vi "Dashboard Main.vi"() -> ()   [LabVIEW 2019]
uses:
  <vilib>/event_ctls.llb/eventvkey.ctl
  <vilib>/Rock Robotics/WPI/Dashboard/WPI_DashboardLogging Global.vi
  <vilib>/Utility/miscctls.llb/LVRowAndColumnTypeDef.ctl
  UnderControl2020/Corsair_V2/Team Code/MotorsGlobal.vi
  UnderControl2020/Corsair_V1/Team Code/Climber Routine.ctl
  <vilib>/Rock Robotics/Network Tables/NT Read Boolean.vi
  UnderControl2020/Corsair_V2/Team Code/JoysticksGlobal.vi
  <vilib>/Rock Robotics/Network Tables/NT Read Numeric Array.vi
  <vilib>/Rock Robotics/Network Tables/NT Read Variant.vi
panel:
  in  "Camera Settings Right":T1={"Frame Rate"=30, "Compression"=30, "Size"=1, "DB Camera Config"=FALSE} {"Frame Rate" scale=1.0..30.0; "Compression" scale=100.0..-1.0; "Size" items=["640x480", "320x240", "160x120"]}
  in  "Camera Name Right":string(combo)="No Camera Selection"
  out "Camera Perf":string
  in  "Camera Settings":T1={"Frame Rate"=30, "Compression"=30, "Size"=1, "DB Camera Config"=FALSE} {"Frame Rate" scale=1.0..30.0; "Compression" scale=100.0..-1.0; "Size" items=["640x480", "320x240", "160x120"]}
  in  "TCP":refnum<k5>
  in  "Rec Mode":enum32{"Stop", "Record", "Playback"}(radio)
  out "Robot IP":string
  out "Image Message":string="Timeout in Camera Communications"
  in  "Dashboard Tab":T2(tab)
  in  "Select Auto":string(combo)="Select Autonomous ..."
  out "NT Connection":bool
  out "MotorChart R":cluster{"Numeric":dbl, "Numeric":dbl}(graph)
  out "MotorChart L":cluster{"Numeric":dbl, "Numeric":dbl}(graph)
  out "MotorSliders R":cluster{"MotorSlide1":dbl, "MotorSlide2":dbl} {"MotorSlide2" scale=-1.0..1.0 scale format="%#_2e"; "MotorSlide1" scale=-1.0..1.0 scale format="%#_2e"}
  out "MotorSliders L":cluster{"MotorSlide1":dbl, "MotorSlide2":dbl} {"MotorSlide2" scale=-1.0..1.0 scale format="%#_2e"; "MotorSlide1" scale=-1.0..1.0 scale format="%#_2e"}
  out "Gyro":dbl(knob) scale=0.0..360.0
  out "JS1 Z":dbl(slide) scale=-1.0..1.0 scale format="%#_2e"
  out "JS1 Graph":cluster{"X":dbl, "Y":dbl}[](graph)
  out "JS1 Buttons":T3
  out "JS2 Z":dbl(slide) scale=-1.0..1.0 scale format="%#_2e"
  out "JS2 Graph":cluster{"X":dbl, "Y":dbl}[](graph)
  out "JS2 Buttons":T3
  out "Mode":T4(ring)=enum."Auto Disabled"
  out "Right Camera Perf":cluster{"Bandwidth (Mbps)":dbl, "FPS":dbl}
  out "Intake on?":bool
  out "LL Valid Target?":bool
  out "Conveyor IR":bool
  out "Climber on?":bool
  out "PTO activated?":bool
  out "Shooter Mode":string
  out "Limelight X":dbl
  out "LimelightY":dbl
  out "Pra qual lado?":string
  out "Camera Image Right":T5(plugin-control)
  in  "DB/String 9":string
  in  "DB/String 8":string
  in  "DB/String 7":string
  in  "DB/String 6":string
  in  "DB/String 5":string
  in  "DB/String 4":string
  in  "DB/String 3":string
  in  "DB/String 2":string
  in  "DB/String 1":string
  in  "DB/String 0":string
  in  "DB/Slider 0":dbl(slide) scale=0.0..5.0
  in  "DB/Slider 1":dbl(slide) scale=0.0..5.0
  in  "DB/Slider 2":dbl(slide) scale=0.0..5.0
  in  "DB/Slider 3":dbl(slide) scale=0.0..5.0
  out "DB/LED 3":bool
  out "DB/LED 2":bool
  out "DB/LED 1":bool
  out "DB/LED 0":bool
  in  "DB/Button 3":bool
  in  "DB/Button 2":bool
  in  "DB/Button 1":bool
  in  "DB/Button 0":bool caption="New Name"
  out "LL Valid Target?.":bool
  out "FlywheelSetpoint":dbl
  out "Reset Encoder":bool
  out "LL in Range?":bool
  out "ClimberSolenoid":bool
  out "LL Mode":dbl
  out "LL LED Status":dbl
  out "TurretEncoder":dbl
  out "RollerOutput":dbl
  out "ConveyorRight\nOutput":dbl
  out "CoveyorLeft\nOutput":dbl
  out "ConveyorMid\nOutput":dbl
  out "IntakeOutput":dbl
  out "ClimberOutput":dbl
  out "Climber on?.":bool
  out "Limelight X 2":dbl
  out "LimelightY 2":dbl
  out "PTO activated?.":bool
  out "Conveyor IR.":bool
  out "Intake on?.":bool
  out "Rumble":dbl
  out "Shooter Mode.":string
  in  "Test Slider":dbl(slide) scale=0.0..100.0 scale format="%#_3g"
  in  "On/Off":bool caption="Solenoid"
  in  "Test Name":u16(ring) items=["Select the test to run..."]
  in  "Test Tree":string(tree)
  in  "Motor":cluster{"Value":dbl, "Enable":bool} {"Value" scale=-1.0..1.0 scale format="%#_3g"}
  out "Progress":T6 {"Test Progress" scale=0.0..100.0}
  in  "Rev/Fwd":cluster{"Forward":bool, "Reverse":bool}
  in  "Test Ring":u16(ring) items=["Monochrome", "Color"]
  out "Cmd Status":string
  in  "Execute Command":bool
  in  "Command Params":string[][](table)
  in  "Command Selection":i32(listbox)
  in  "CheckList":i32(listbox)
  out "Tree":string(tree)
  out "Camera Image":T5(plugin-control)
  in  "Camera Name":string(combo)="No Camera Selection"
  # "HW"
  # "HW"
  # "Drive Motors"
  # "Joysticks"
  # "Front"
  # "Left"
  # "Back"
  # "Shooter"
  # "Conveyor and intake"
  # "Climber"
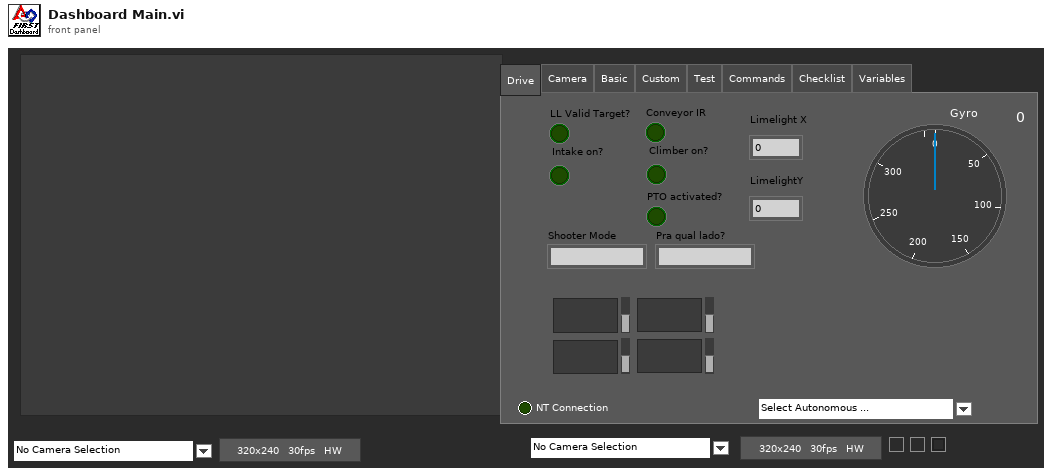
[diagram p1: front panel]
types:
  T1 = cluster{"Frame Rate":i32, "Compression":i32, "Size":u16, "DB Camera Config":bool}
  T2 = enum32{"Drive", "Camera", "Basic", "Custom", "Test", "Commands", "Checklist", "Variables"}
  T3 = cluster{bool, bool, bool, bool, bool, bool, bool, bool, bool, bool, bool, bool}
  T4 = enum8{"Tele-Op Disabled", "Tele-Op Enabled", "Auto Disabled", "Auto Enabled", "Test Disabled", "Test Enabled", "Disconnected", "No Code", "E-Stop"}
  T5 = typedef "IMAQ Image.ctl" = refnum<image>
  T6 = cluster{"Test Progress":u8, "Test Progress Text":string}
  T7 = cluster{"Save Path":path, "Interval (s)":dbl, "Keep":i32}
  T8 = typedef "Image Type" = u32
  T9 = cluster{"IDs":cluster{"RPC field ID":u16, "Unique ID":u16}, "String":string}
  T10 = typedef "Climber Routine.ctl" = enum16{"Standart", "Vibrate *Lenny Face*", "Open da Boi", "Engage on the Bar!", "Pull Our Hope", "Deu por Hoje"}
  T11 = cluster{"Error Strings":string, "Disable Counts":cluster{u16, u16}, "Rail Faults":cluster{u16, u16, u16}, "Robot IP":string, "DB Mode":u8, "Event Info":cluster{"Name":string, "Type":u8, "Number":u16, "Replay":u8}}
  T12 = cluster{"Storage":cluster{"Disk Free":u64, "RAM Block":u32, "RAM free":u32}, "CPU Utilization":cluster{"CPU % ISR":sgl, "CPU % Time Crit":sgl, "CPU % Timed Str":sgl, "CPU % High":sgl, "CPU % Above":sgl, "CPU % Normal":sgl, "CPU % Low":sgl}, "CAN":cluster{"% Bus Utilization":sgl, "Bus Off Cnt":u32, "TX_FIFO Full Cnt":u32, "Receive Error Cnt":u8, "Transmit Error Cnt":u8}, "HID":cluster{"HID Outputs":u32, "Rumble Low":u16, "Rumble High":u16}[]}
  T13 = cluster{"Status bits":cluster{"Test Mode":bool, "Autonomous":bool, "Enabled":bool, "Code Start":bool, "Brownout":bool, "Reserved 2":bool, "Reserved 3":bool, "E-Stop":bool}, "Code Trace":cluster{"Disabled":bool, "TeleOp":bool, "Auto":bool, "Test":bool}, "Controller Type":enum16{"unknown", "cRIO", "roboRio"}, "Code?":enum16{"unknown", "noCode", "code"}, "Battery V":dbl}
  T14 = cluster{"Control Bits":cluster{"TestMode":bool, "Autonomous":bool, "Enabled":bool, "FMS Present":bool, bool, bool, bool, "E-Stop":bool}, "Team Station ":u8, "Countdown":sgl, "Joystick Values":cluster{"Axes":dbl[], "Buttons":bool[], "POVs":i16[]}[]}
  T15 = cluster{"Axes":dbl[], "Buttons":bool[], "POVs":i16[]}[]
  T16 = cluster{"Axes":dbl[], "Buttons":bool[], "POVs":i16[]}
  T17 = cluster{"Buttons[0]":bool, "Buttons[1]":bool, "Buttons[2]":bool, "Buttons[3]":bool, "Buttons[4]":bool, "Buttons[5]":bool, "Buttons[6]":bool, "Buttons[7]":bool, "Buttons[8]":bool, "Buttons[9]":bool, "Buttons[10]":bool, "Buttons[11]":bool}
  T18 = cluster{"Camera Image":refnum<vi>, "Dashboard Tab":refnum<vi>, void, "Rec Mode":refnum<vi>, "Test Slider":refnum<vi>, "On/Off ":refnum<vi>, "Test Ring":refnum<vi>, "Rev/Fwd":refnum<vi>, "Test Name":refnum<vi>, "Motor":refnum<vi>, "Progress":refnum<vi>, "CheckList":refnum<vi>, "Tree":refnum<vi>, "Test Tree":refnum<vi>, "Command Params":refnum<vi>, "Command Selection":refnum<vi>, "Execute Command":refnum<vi>, "Cmd Status":refnum<vi>, "Camera Settings":refnum<vi>, "Camera Name":refnum<vi>, "Camera Perf":refnum<vi>, "Camera Settings Right":refnum<vi>, "Camera Name Right":refnum<vi>, "Camera Image Right":refnum<vi>}
  T19 = cluster{"Global Rectangle":i32[], "Contours":cluster{"Contour Type":u32, "ROI Type":u32, "Points":i32[]}[]}
  T20 = cluster{"Camera Name":string, string, "Saved DB Images Info":cluster{"Save Path":path, "Interval (s)":dbl, "Keep":i32}}
  T21 = cluster{"Camera Name Right":string, string, "Saved DB Images Info":cluster{"Save Path":path, "Interval (s)":dbl, "Keep":i32}}
  T22 = cluster{"Operation":enum16{"Update", "Clear"}, "Color Box":u32}[]
  T23 = typedef "eventvkey.ctl" = enum16{"ASCII", "Enter", "Return", "Shift", "Ctrl", "Alt", "Cmd", "Opt", "Caps", "NumLock", "Clear", "Break", "Up", "Down", "Left", "Right", "Insert", "Delete", "Home", "End", "PageUp", "PageDown", "Escape", "Help", "Pause", "ScrollLock", "F1", "F2", "F3", "F4", "F5", "F6", "F7", "F8", "F9", "F10", "F11", "F12", "F13", "F14", "F15", "F16", "F17", "F18", "F19", "F20", "F21", "F22", "F23", "F24", "Play", "VolumeUp", "VolumeDown", "Mute", "Two Byte Char"}
  T24 = cluster{"Image Size":bool, "Image Type":bool, "Pixel Value":bool, "ROI Information":bool, "Zoom Factor":bool}
  T25 = cluster{"Operation":enum16{"Update", "Clear"}, "Color Box":u32}
  T26 = typedef "LVRowAndColumnTypeDef.ctl" = cluster{"Row":i32, "Column":i32}
  T27 = cluster{"Shift":bool, "Ctrl":bool, "Alt":bool, "Cmd":bool, "Opt":bool}
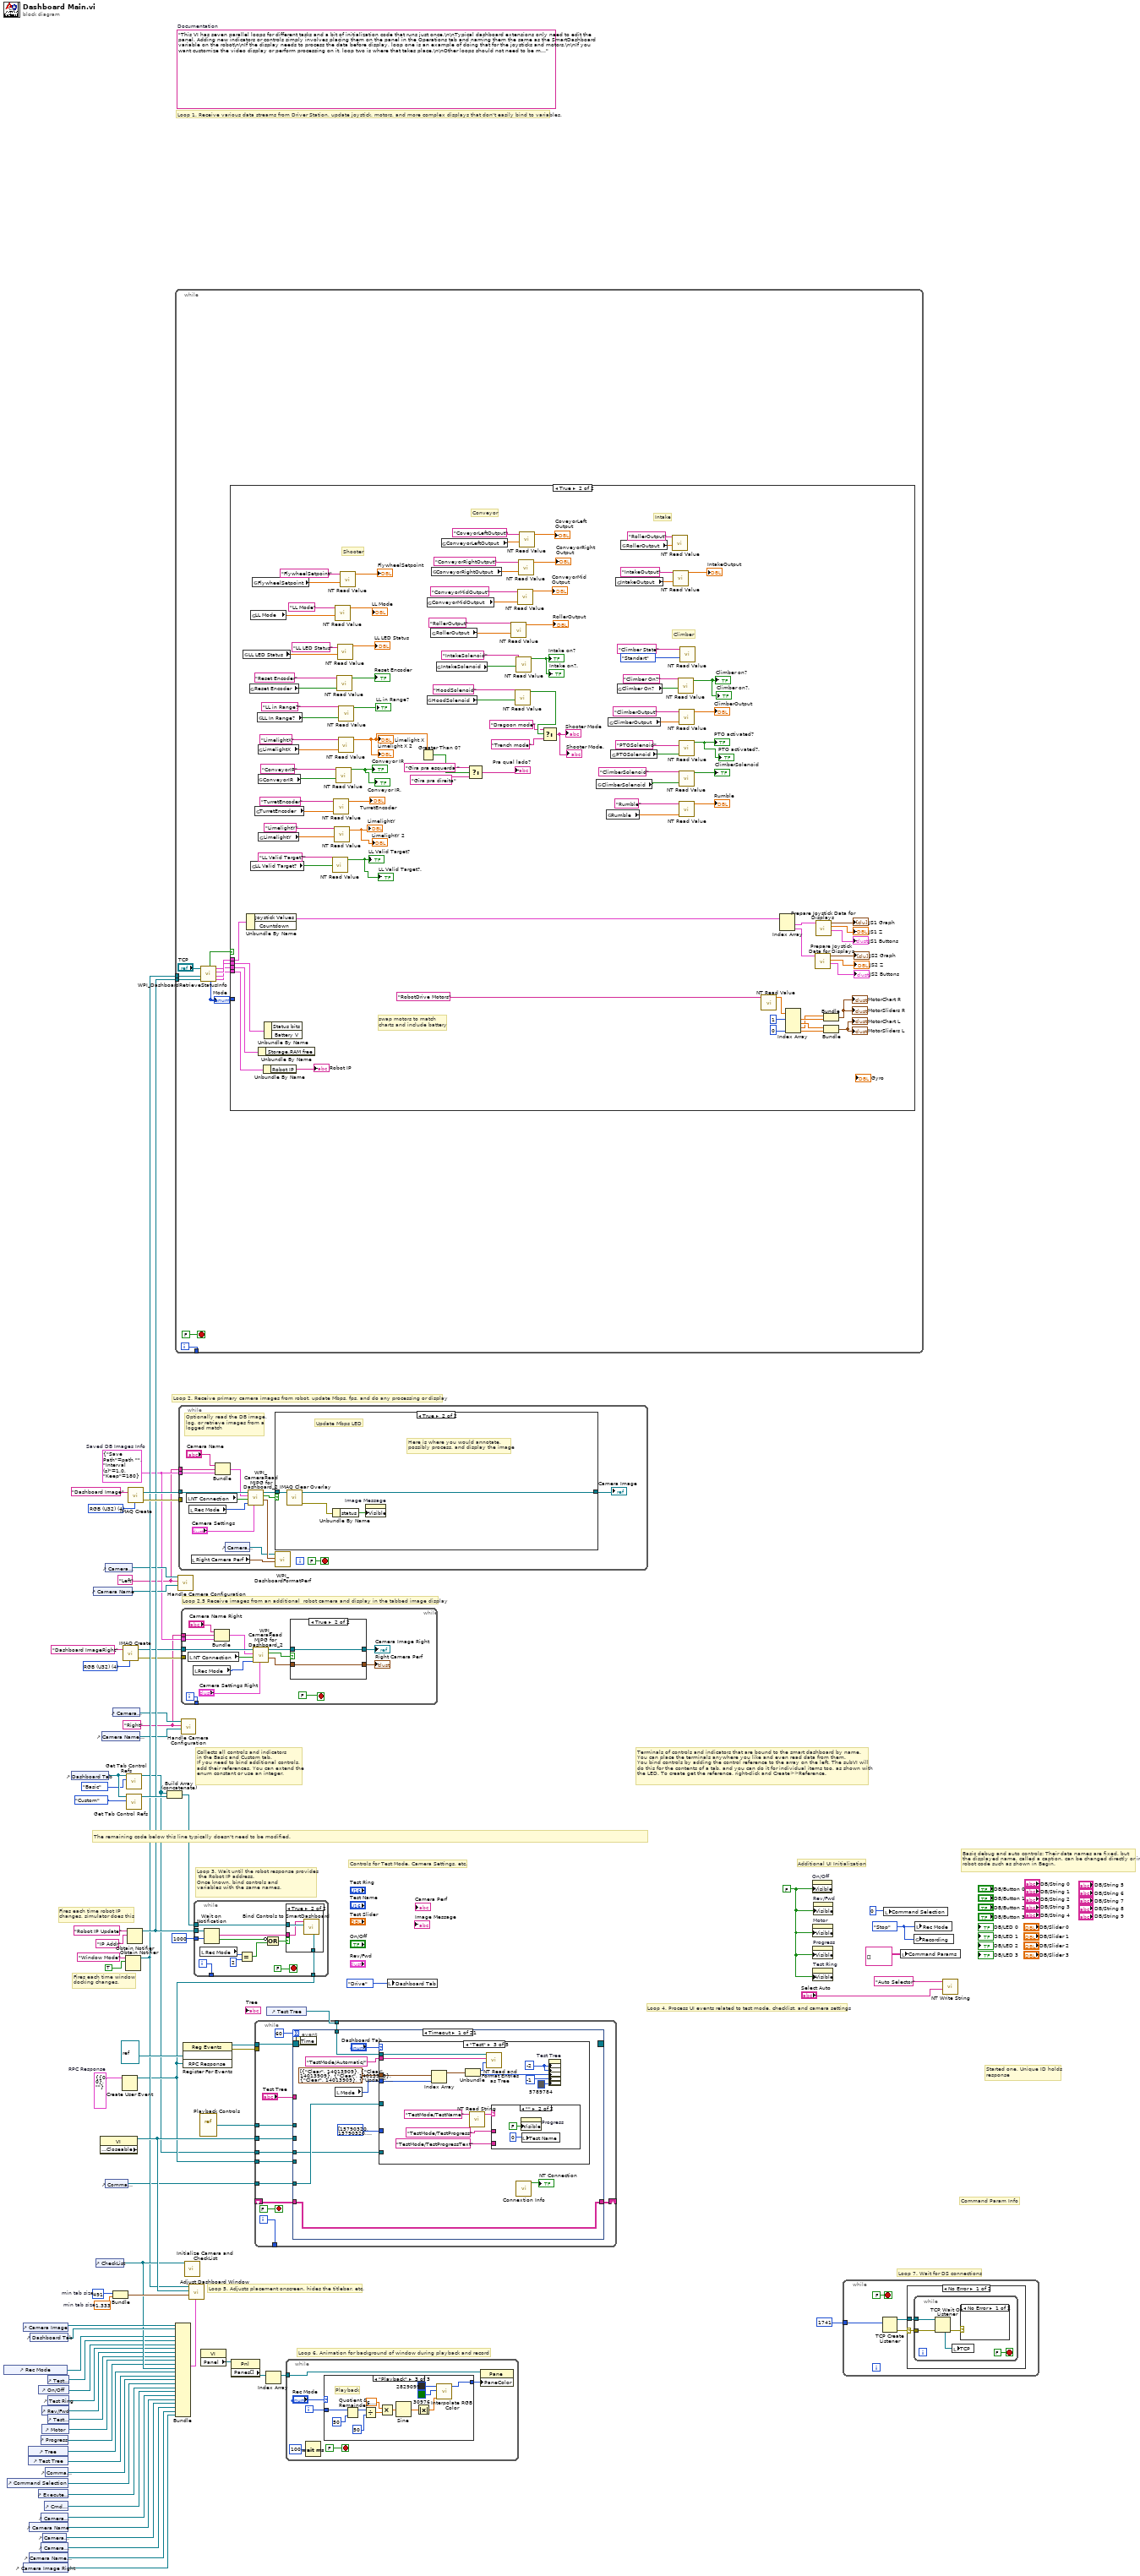
[diagram p0: block diagram]
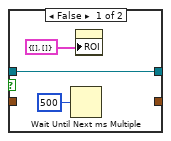
[diagram p2: hidden frame]
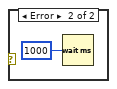
[diagram p3: hidden frame]
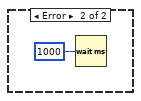
[diagram p4: hidden frame]
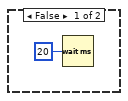
[diagram p5: hidden frame]
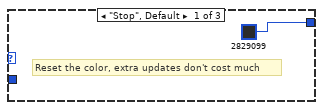
[diagram p6: hidden frame]
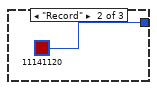
[diagram p7: hidden frame]
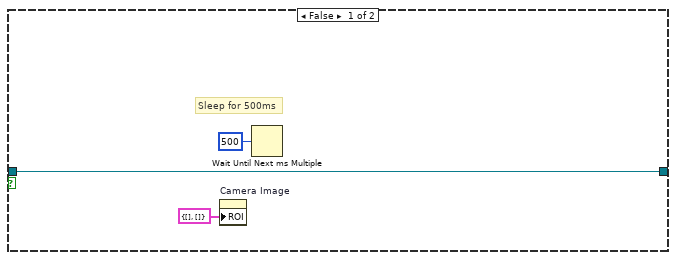
[diagram p9: hidden frame]
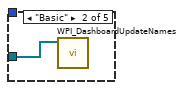
[diagram p11: hidden frame]
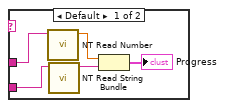
[diagram p12: hidden frame]
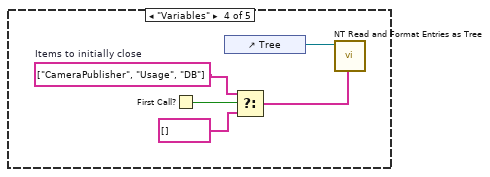
[diagram p13: hidden frame]
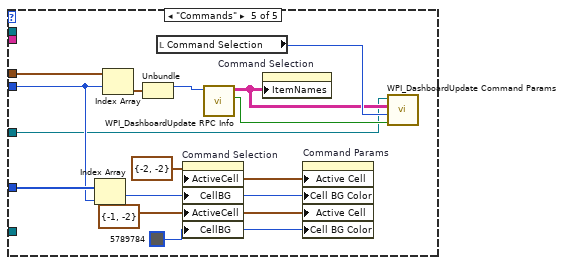
[diagram p14: hidden frame]
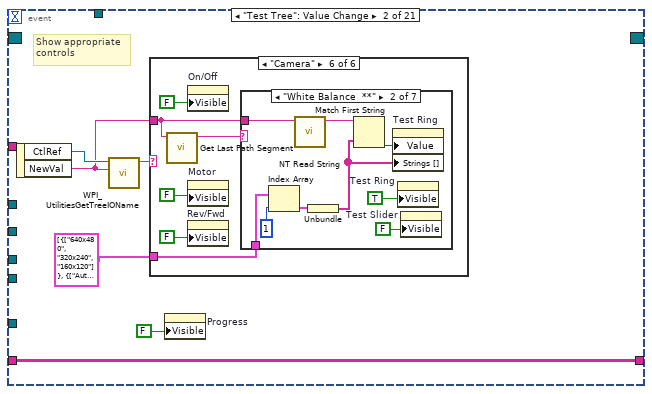
[diagram p15: hidden frame]
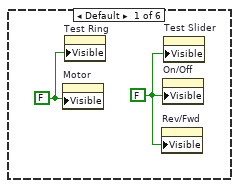
[diagram p16: hidden frame]
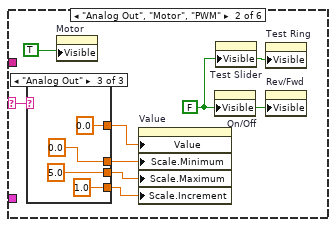
[diagram p17: hidden frame]
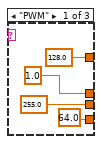
[diagram p18: hidden frame]
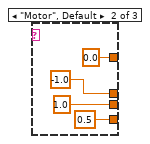
[diagram p19: hidden frame]
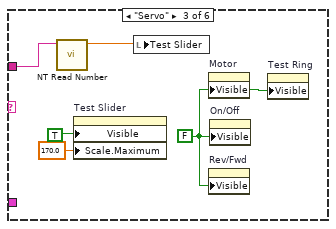
[diagram p20: hidden frame]
diagram:
  w3 = T7 {"Save Path"=path "", "Interval (s)"=1.0, "Keep"=180}  # Saved DB Images Info
  w2 = "Right"
  w1 = "Left"
  w13 = T8 4 items=["Grayscale (U8)", "Grayscale (I16)", "Grayscale (SGL)", "Complex (CSG)", "RGB (U32)", "HSL (U32)", "RGB (U64)"] ("Image Type")
  w29 = T9 {"IDs"={"RPC field ID"=0, "Unique ID"=0}, "String"=""}  # RPC Response
  w52 = 491  # min tab size
  w51 = 1.333  # min tab size
  w59 = enum32{"Stop", "Record", "Playback"}."Stop" ("Rec Mode")
  w36 = FALSE ("Visible")
  (unwired) "This VI has seven parallel loops for different tasks and a bit of initialization code that runs just once.\n\nTypical dashboard extensions only need to edit the panel. Adding new indicators or controls simply involves placing them on the panel in the Operations tab and naming them the same as the SmartDashboard variable on the robot\n\nIf the display needs to process the data before display, loop one is an example of doing that for the joysticks and motors.\n\nIf you want customize the video display or perform processing on it, loop two is where that takes place.\n\nOther loops should not need to be modified. They are pretty standard, and document the task they perform."  # Documentation
  w76 = T8 4 items=["Grayscale (U8)", "Grayscale (I16)", "Grayscale (SGL)", "Complex (CSG)", "RGB (U32)", "HSL (U32)", "RGB (U64)"] ("Image Type")
  # "Loop 2.5 Receive images from an additional  robot camera and display in the tabbed image display"
  # "Command Param Info"
  # "Started one, Unique ID holds\nresponse"
  # "Loop 7. Wait for DS connections"
  # "Basic debug and auto controls: Their data names are fixed, but\nthe displayed name, called a caption, can be changed directly or in\nrobot code such as shown in Begin."
  # "Controls for Test Mode, Camera Settings, etc."
  # "Additional UI Initialization"
  # "Loop 6. Animation for background of window during playback and record"
  # "Fires each time robot IP\nchanges, simulator does this"
  # "Fires each time window\ndocking changes."
  # "Collects all controls and indicators\nin the Basic and Custom tab.\nIf you need to bind additional controls,\nadd their references. You can extend the\nenum constant or use an integer."
  # "The remaining code below this line typically doesn't need to be modified."
  # "Loop 4. Process UI events related to test mode, checklist, and camera settings"
  # "Terminals of controls and indicators that are bound to the smart dashboard by name.\nYou can place the terminals anywhere you like and even read data from them.\nYou bind controls by adding the control reference to the array on the left. The subVI will\ndo this for the contents of a tab, and you can do it for individual items too, as shown with\nthe LED. To create get the reference, right-click and Create>>Reference."
  # "Loop 3. Wait until the robot response provides\n the Robot IP address.\nOnce known, bind controls and\nvariables with the same names."
  # "Loop 5. Adjusts placement onscreen, hides the titlebar, etc."
  # "Loop 1. Receive various data streams from Driver Station, update joystick, motors, and more complex displays that don't easily bind to variables."
  # "Loop 2. Receive primary camera images from robot, update Mbps, fps, and do any processing or display"
  n1 = control-ref of="Rec Mode"() -> (w42:refnum<vi>)
  n2 = control-ref of="Command Selection"() -> (w28:refnum<vi>)
  n3 = control-ref of="Camera Image Right"() -> (w6:refnum<vi>)
  n4 = control-ref of="Camera Image"() -> (w54:refnum<vi>)
  n5 = control-ref of="Tree"() -> (w46:refnum<vi>)
  n6 = control-ref of="Test Tree"() -> (w45:refnum<vi>)
  n7 = control-ref of="Camera Name"() -> (w19:refnum<vi>)
  n8 = control-ref of="Camera Name Right"() -> (w7:refnum<vi>)
  n9 = control-ref of="Dashboard Tab"() -> (w53:refnum<vi>)
  n10 = control-ref of="Execute Command"() -> (w30:refnum<vi>)
  n11 = control-ref of="On/Off"() -> (w40:refnum<vi>)
  n12 = control-ref of="Progress"() -> (w37:refnum<vi>)
  n13 = control-ref of="Camera Settings"() -> (w20:refnum<vi>)
  n14 = control-ref of="Camera Settings Right"() -> (w8:refnum<vi>)
  n15 = control-ref of="Rev/Fwd"() -> (w38:refnum<vi>)
  n16 = control-ref of="Motor"() -> (w43:refnum<vi>)
  n17 = control-ref of="Camera Perf"() -> (w18:refnum<vi>)
  n18 = control-ref of="Cmd Status"() -> (w24:refnum<vi>)
  n19 = control-ref of="Command Params"() -> (w31:refnum<vi>)
  n20 = control-ref of="Test Slider"() -> (w41:refnum<vi>)
  n21 = control-ref of="Test Ring"() -> (w39:refnum<vi>)
  n22 = control-ref of="Test Name"() -> (w44:refnum<vi>)
  n23 = control-ref of="Dashboard Tab"() -> (w57:refnum<vi>)
  n24 = control-ref of="Camera Name"() -> (w21:refnum<vi>)
  n25 = control-ref of="CheckList"() -> (w47:refnum<vi>)
  n26 = property class="VI" props=["Front Panel.Closeable"]() -> (reference out=w58:refnum<vi>)  [unwired: 2 in, 2 out]
  n27 = control-ref of="Camera Name Right"() -> (w9:refnum<vi>)
  n28 = control-ref of="Camera Settings"() -> (w22:refnum<vi>)
  n29 = control-ref of="Command Params"() -> (w23:refnum<vi>)
  n30 = control-ref of="Camera Settings Right"() -> (w10:refnum<vi>)
  n31 = Bundle("min tab size"=w52, "min tab size"=w51) -> (w50:cluster{"min tab size":i32, "min tab size":dbl})  [unwired: 1 in]
  n32 = Create User Event(user event datatype=w29) -> (user event=w25:refnum<user-event>)  [unwired: 1 in, 1 out]
  n33 = call "IMAQ Create"("Image Name"="Dashboard ImageRight", "Image Type"=w13) -> ("New Image"=w12:T5, "error out"=w11:errorcluster)  [unwired: 2 in, 1 out]
  n34 = Obtain Notifier(name (unnamed)="Window Mode", notification data type=TRUE) -> (notifier out=w34:refnum<notifier>)  [unwired: 2 in, 2 out]
  n35 = call <vilib>:"Get Tab Control Refs.vi"("Page Index"=T2."Basic" ("Dashboard Tab"), "TabControl in"=w57) -> ("ControlsOnPage"=w17:refnum<vi>[])  [unwired: 9 in]
  n36 = call <vilib>:"Get Tab Control Refs.vi"("Page Index"=T2."Custom" ("Dashboard Tab"), "TabControl in"=w57) -> ("ControlsOnPage"=w56:refnum<vi>[])  [unwired: 9 in]
  n37 = Obtain Notifier(name (unnamed)="Robot IP Update", notification data type="IP Addr" ("name (unnamed)")) -> (notifier out=w35:refnum<notifier>)  [unwired: 2 in, 2 out]
  n38 = call "IMAQ Create"("Image Name"="Dashboard Image", "Image Type"=w76) -> ("New Image"=w74:T5, "error out"=w73:errorcluster)  [unwired: 2 in, 1 out]
  n39 = Build Array (concatenate)(w17, w56) -> (w55:refnum<vi>[])
  n40 = while {
    tunnel: [w86] -> _
    tunnel: w35 -> [w80]
    tunnel: w34 -> [w77]
    i -> [w86]
    stop <- FALSE stop-if-true
    n41 = call <vilib>:"WPI_DashboardRetrieveStatusInfo.vi"("Binding Refnum"=w80, "Window Mode Notifier"=w77, "TCP Cnx"="TCP") -> ("Power and Errors"=w81:T11, "Robot Metrics"=w84:T12, "Status Info"=w85:T13, "Control Info"=w82:T14, "Robot Mode"=w79:T4, "Process?"=w83:bool)  [unwired: 3 in]
    "Mode" <- w79
    n42 = case shown="True" w83 {
      tunnel: w85 -> [_ w189]
      tunnel: w84 -> [_ w188]
      tunnel: w82 -> [_ w187]
      tunnel: w81 -> [_ w186]
      tunnel: w79 -> [_ _]
      frame False {
        n43 = Wait (ms)(milliseconds to wait=u32 20) -> ()  [unwired: 1 out]
      }
      frame True {
        # "Climber"
        # "Intake"
        # "Conveyor"
        # "Shooter"
        # "swap motors to match\ncharts and include battery"
        n44 = global read "MotorsGlobal.vi" "LL LED Status"() -> (w162:dbl)
        n45 = Unbundle By Name(w187) -> ("Joystick Values"=w177:T15)  [unwired: 1 out]
        n46 = global read "MotorsGlobal.vi" "Reset Encoder"() -> (w142:bool)
        n47 = global read "MotorsGlobal.vi" "LL Mode"() -> (w163:dbl)
        n48 = global read "MotorsGlobal.vi" "LL Valid Target?"() -> (w119:bool)
        n49 = global read "MotorsGlobal.vi" "FlywheelSetpoint"() -> (w165:dbl)
        n50 = global read "MotorsGlobal.vi" "TurretEncoder"() -> (w123:dbl)
        n51 = global read "MotorsGlobal.vi" "LL In Range?"() -> (w129:bool)
        n52 = global read "MotorsGlobal.vi" "LimelightX"() -> (w127:dbl)
        n53 = global read "MotorsGlobal.vi" "ConveyorIR"() -> (w125:bool)
        n54 = global read "MotorsGlobal.vi" "LimelightY"() -> (w121:dbl)
        n55 = Unbundle By Name(w188) -> ()  [unwired: 1 out]
        n56 = Unbundle By Name(w186) -> ("Robot IP"=→"Robot IP":string)
        n57 = Unbundle By Name(w189) -> ()  [unwired: 2 out]
        n58 = call-poly <vilib>:"NT Read Value.vi"("Default Value"=w119, "Name"="LL Valid Target?") -> ("Boolean"=→"LL Valid Target?" →"LL Valid Target?.":bool)  [unwired: 8 in, 1 out]
        n59 = call-poly <vilib>:"NT Read Value.vi"("Default Value"=w123, "Name"="TurretEncoder") -> ("Numeric"=→"TurretEncoder":dbl)  [unwired: 8 in, 1 out]
        n60 = call-poly <vilib>:"NT Read Value.vi"("Default Value"=w121, "Name"="LimelightY") -> ("Numeric"=→"LimelightY" →"LimelightY 2":dbl)  [unwired: 8 in, 1 out]
        n61 = call-poly <vilib>:"NT Read Value.vi"("Default Value"=w163, "Name"="LL Mode") -> ("Numeric"=→"LL Mode":dbl)  [unwired: 8 in, 1 out]
        n62 = call-poly <vilib>:"NT Read Value.vi"("Default Value"=w125, "Name"="ConveyorIR") -> ("Boolean"=→"Conveyor IR" →"Conveyor IR.":bool)  [unwired: 8 in, 1 out]
        n63 = call-poly <vilib>:"NT Read Value.vi"("Default Value"=w142, "Name"="Reset Encoder") -> ("Boolean"=→"Reset Encoder":bool)  [unwired: 8 in, 1 out]
        n64 = call-poly <vilib>:"NT Read Value.vi"("Default Value"=w162, "Name"="LL LED Status") -> ("Numeric"=→"LL LED Status":dbl)  [unwired: 8 in, 1 out]
        n65 = call-poly <vilib>:"NT Read Value.vi"("Default Value"=w127, "Name"="LimelightX") -> ("Numeric"=w93:dbl)  [unwired: 8 in, 1 out]
        "Limelight X" <- w93
        "Limelight X 2" <- w93
        n66 = call-poly <vilib>:"NT Read Value.vi"("Default Value"=w129, "Name"="LL in Range?") -> ("Boolean"=→"LL in Range?":bool)  [unwired: 8 in, 1 out]
        n67 = call-poly <vilib>:"NT Read Value.vi"("Default Value"=w165, "Name"="FlywheelSetpoint") -> ("Numeric"=→"FlywheelSetpoint":dbl)  [unwired: 8 in, 1 out]
        n68 = Greater Than 0?(x=w93) -> (x > 0?=w92:bool)
        n69 = global read "MotorsGlobal.vi" "ConveyorMidOutput"() -> (w153:dbl)
        n70 = global read "MotorsGlobal.vi" "HoodSolenoid"() -> (w144:bool)
        n71 = global read "MotorsGlobal.vi" "RollerOutput"() -> (w151:dbl)
        n72 = global read "MotorsGlobal.vi" "ConveyorRightOutput"() -> (w155:dbl)
        n73 = global read "MotorsGlobal.vi" "IntakeSolenoid"() -> (w146:bool)
        n74 = global read "MotorsGlobal.vi" "ConveyorLeftOutput"() -> (w157:dbl)
        n75 = Select(t="Gira pra esquerda ", s=w92, f="Gira pra direita") -> (s? t:f=→"Pra qual lado?":string)
        n76 = call-poly <vilib>:"NT Read Value.vi"("Default Value"=w151, "Name"="RollerOutput") -> ("Numeric"=→"RollerOutput":dbl)  [unwired: 8 in, 1 out]
        n77 = call-poly <vilib>:"NT Read Value.vi"("Default Value"=w144, "Name"="HoodSolenoid") -> ("Boolean"=w117:bool)  [unwired: 8 in, 1 out]
        n78 = call-poly <vilib>:"NT Read Value.vi"("Default Value"=w146, "Name"="IntakeSolenoid") -> ("Boolean"=→"Intake on?" →"Intake on?.":bool)  [unwired: 8 in, 1 out]
        n79 = call-poly <vilib>:"NT Read Value.vi"("Default Value"=w153, "Name"="ConveyorMidOutput") -> ("Numeric"=→"ConveyorMid\nOutput":dbl)  [unwired: 8 in, 1 out]
        n80 = call-poly <vilib>:"NT Read Value.vi"("Default Value"=w155, "Name"="ConveyorRightOutput") -> ("Numeric"=→"ConveyorRight\nOutput":dbl)  [unwired: 8 in, 1 out]
        n81 = call-poly <vilib>:"NT Read Value.vi"("Default Value"=w157, "Name"="CoveyorLeftOutput") -> ("Numeric"=→"CoveyorLeft\nOutput":dbl)  [unwired: 8 in, 1 out]
        n82 = Select(t="Dragoon mode", s=w117, f="Trench mode") -> (s? t:f=→"Shooter Mode" →"Shooter Mode.":string)
        n83 = global read "MotorsGlobal.vi" "ClimberSolenoid"() -> (w131:bool)
        n84 = global read "JoysticksGlobal.vi" "Rumble"() -> (w133:dbl)
        n85 = global read "MotorsGlobal.vi" "ClimberOutput"() -> (w137:dbl)
        n86 = global read "MotorsGlobal.vi" "PTOSolenoid"() -> (w135:bool)
        n87 = global read "MotorsGlobal.vi" "IntakeOutput"() -> (w159:dbl)
        n88 = global read "MotorsGlobal.vi" "Climber On?"() -> (w139:bool)
        n89 = global read "MotorsGlobal.vi" "RollerOutput"() -> (w147:dbl)
        n90 = call-poly <vilib>:"NT Read Value.vi"("Default Value"=w147, "Name"="RollerOutput") -> ()  [unwired: 8 in, 2 out]
        n91 = call-poly <vilib>:"NT Read Value.vi"("Default Value"=w159, "Name"="IntakeOutput") -> ("Numeric"=→"IntakeOutput":dbl)  [unwired: 8 in, 1 out]
        n92 = call-poly <vilib>:"NT Read Value.vi"("Default Value"=w139, "Name"="Climber On?") -> ("Boolean"=→"Climber on?" →"Climber on?.":bool)  [unwired: 8 in, 1 out]
        n93 = call-poly <vilib>:"NT Read Value.vi"("Default Value"=w131, "Name"="ClimberSolenoid") -> ("Boolean"=→"ClimberSolenoid":bool)  [unwired: 8 in, 1 out]
        n94 = call-poly <vilib>:"NT Read Value.vi"("Default Value"=w137, "Name"="ClimberOutput") -> ("Numeric"=→"ClimberOutput":dbl)  [unwired: 8 in, 1 out]
        n95 = call-poly <vilib>:"NT Read Value.vi"("Default Value"=w135, "Name"="PTOSolenoid") -> ("Boolean"=→"PTO activated?" →"PTO activated?.":bool)  [unwired: 8 in, 1 out]
        n96 = call-poly <vilib>:"NT Read Value.vi"("Default Value"=w133, "Name"="Rumble") -> ("Numeric"=→"Rumble":dbl)  [unwired: 8 in, 1 out]
        n97 = call-poly <vilib>:"NT Read Value.vi"("Default Value"=Climber_Routine."Standart", "Name"="Climber State") -> ()  [unwired: 8 in, 2 out]
        n98 = call-poly <vilib>:"NT Read Value.vi"("Name"="RobotDrive Motors") -> ("Numeric Array"=w167:dbl[])  [unwired: 9 in, 1 out]
        n99 = Index Array(array=w177) -> (element #1=w176:T16, element #2=w172:T16)  [unwired: 2 in]
        n100 = Index Array(array=w167, index #1=1, index #4=0) -> (element #1=w181:dbl, element #2=w182:dbl, element #3=w180:dbl, element #4=w185:dbl)  [unwired: 2 in]
        n101 = call "Prepare Joystick Data for Displays.vi"("Joystick Values"=w172) -> ("Buttons"=→"JS2 Buttons":T17, "Z Axis"=→"JS2 Z":dbl, "Cartesian Data"=→"JS2 Graph":cluster{"X axis":dbl, "X axis":dbl}[])  [unwired: 8 in]
        n102 = call "Prepare Joystick Data for Displays.vi"("Joystick Values"=w176) -> ("Buttons"=→"JS1 Buttons":T17, "Z Axis"=→"JS1 Z":dbl, "Cartesian Data"=→"JS1 Graph":cluster{"X axis":dbl, "X axis":dbl}[])  [unwired: 8 in]
        n103 = Bundle("Numeric"=w180, "Numeric"=w181) -> (→"MotorChart R" →"MotorSliders R":cluster{"Numeric":dbl, "Numeric":dbl})  [unwired: 1 in]
        n104 = Bundle("Numeric"=w182, "Numeric"=w185) -> (→"MotorChart L" →"MotorSliders L":cluster{"Numeric":dbl, "Numeric":dbl})  [unwired: 1 in]
      }
    }
  }
  n105 = Bundle("Camera Image"=w54, "Dashboard Tab"=w53, "Rec Mode"=w42, "Test Slider"=w41, "On/Off"=w40, "Test Ring"=w39, "Rev/Fwd"=w38, "Test Name"=w44, "Motor"=w43, "Progress"=w37, "CheckList"=w47, "Tree"=w46, "Test Tree"=w45, "Command Params"=w31, "Command Selection"=w28, "Execute Command"=w30, "Cmd Status"=w24, "Camera Settings"=w20, "Camera Name"=w19, "Camera Perf"=w18, "Camera Settings Right"=w8, "Camera Name Right"=w7, "Camera Image Right"=w6) -> (w48:T18, w49)  [unwired: 1 in]
  n106 = call "Handle Camera Configuration.vi"("CameraNameRef"=w21, "Display Name"=w1, "ClusterRef"=w22) -> ()  [unwired: 9 in]
  n107 = while {
    tunnel: w74 -> [w203]
    tunnel: w73 -> [_]
    tunnel: w3 -> [w196]
    tunnel: w1 -> [w193]
    stop <- FALSE stop-if-true
    # "Optionally read the DB image,\nlog, or retrieve images from a\nlogged match"
    n108 = local read "NT Connection"() -> (w197:bool)
    n109 = local read "Rec Mode"() -> (w200:enum32{"Stop", "Record", "Playback"})
    n110 = local read "Right Camera Perf"() -> (w191:cluster{"Bandwidth (Mbps)":dbl, "FPS":dbl})
    n111 = Bundle("Camera Name"="Camera Name", w193, "Saved DB Images Info"=w196) -> (w195:T20)  [unwired: 1 in]
    n112 = control-ref of="Camera Perf"() -> (w190:refnum<vi>)
    n113 = call <vilib>:"WPI_CameraRead MJPG for Dashboard_2.vi"("Camera Settings"="Camera Settings", "Rec Mode"=w200, "NT Connection"=w197, "Capture Info"=w195, "Image in"=w203) -> ("perf info"=w192:cluster{"Bandwidth (Mbps)":dbl, "fps":dbl}, "Active"=w201:bool, "Image\\ out"=w202:T5)  [unwired: 4 in]
    n114 = case shown="True" w201 {
      tunnel: w202 -> [w206 w209]
      tunnel: [w206 w208] -> w198
      frame False {
        # "Sleep for 500ms"
        n115 = property on="Camera Image" class="ImageControl"("ROI"=T19 {"Global Rectangle"=[], "Contours"=[]}) -> ()  [unwired: 2 in, 2 out]
        n116 = Wait Until Next ms Multiple(millisecond multiple=u32 500) -> ()  [unwired: 1 out]
      }
      frame True {
        # "Here is where you would annotate,\npossibly process, and display the image"
        # "Update Mbps LED"
        n117 = call "IMAQ Clear Overlay"("Image"=w209) -> ("error out"=w210:errorcluster, "Image Out"=w208:T5)  [unwired: 2 in, 7 out]
        n118 = Unbundle By Name(w210) -> ("status"=w211:bool)
        n119 = property on="Image Message" class="Str"("Visible"=w211) -> ()  [unwired: 2 in, 2 out]
      }
    }
    "Camera Image" <- w198
    n120 = call <vilib>:"WPI_DashboardFormatPerf.vi"("Right Camera Perf"=w191, "Performance"=w192, "String in"=w190) -> ()  [unwired: 9 in]
  }
  n121 = call "Handle Camera Configuration.vi"("CameraNameRef"=w9, "Display Name"=w2, "ClusterRef"=w10) -> ()  [unwired: 9 in]
  n122 = while {
    tunnel: w12 -> [w226]
    tunnel: w11 -> [_]
    tunnel: [w221] -> _
    tunnel: w3 -> [w217]
    tunnel: w2 -> [w214]
    i -> [w221]
    stop <- FALSE stop-if-true
    n123 = local read "NT Connection"() -> (w218:bool)
    n124 = local read "Rec Mode"() -> (w225:enum32{"Stop", "Record", "Playback"})
    n125 = Bundle("Camera Name Right"="Camera Name Right", w214, "Saved DB Images Info"=w217) -> (w216:T21)  [unwired: 1 in]
    n126 = call <vilib>:"WPI_CameraRead MJPG for Dashboard_2.vi"("Camera Settings"="Camera Settings Right", "Rec Mode"=w225, "NT Connection"=w218, "Capture Info"=w216, "Image in"=w226) -> ("perf info"=w212:cluster{"Bandwidth (Mbps)":dbl, "fps":dbl}, "Active"=w220:bool, "Image\\ out"=w223:T5)  [unwired: 4 in]
    n127 = case shown="True" w220 {
      tunnel: w223 -> [w228 w231]
      tunnel: [w228 w231] -> w219
      tunnel: [_ w230] -> w213
      tunnel: w212 -> [_ w230]
      frame False {
        n128 = Wait Until Next ms Multiple(millisecond multiple=u32 500) -> ()  [unwired: 1 out]
        n129 = property on="Camera Image Right" class="ImageControl"("ROI"=T19 {"Global Rectangle"=[], "Contours"=[]}) -> ()  [unwired: 2 in, 2 out]
      }
      frame True {
      }
    }
    "Camera Image Right" <- w219
    "Right Camera Perf" <- w213
  }
  n130 = register-events(refnum<vi> refnum, w25) -> (reference out=w63:refnum<event-registration>, error out=w62:errorcluster)  [unwired: 2 in]
  n131 = call "Initialize Camera and CheckList.vi"("ListBox in"=w47) -> ()  [unwired: 11 in]
  n132 = call "Adjust Dashboard Window.vi"("Sizing Refnums"=w48, "Size Constraints"=w50, "VI"=w58, "WIn Mode"=w34) -> ()  [unwired: 8 in]
  n133 = while {
    tunnel: w55 -> [w243]
    tunnel: w35 -> [w241]
    tunnel: [w239] -> _
    tunnel: u32 1000 ("milliseconds to wait") -> [w238]
    tunnel: w25 -> [w232]
    i -> [w239]
    stop <- FALSE stop-if-true
    n134 = local read "Rec Mode"() -> (w234:enum32{"Stop", "Record", "Playback"})
    n135 = Wait on Notification(notifier=w241, timeout in ms (-1)=w238) -> (notification=w240:string, timed out?=w236:bool)  [unwired: 2 in, 2 out]
    n136 = Equal?(x=w234, y=u16 2 ("Rec Mode")) -> (x = y?=w235:bool)
    n137 = Compound Arithmetic op=OR(invert w236, w235) -> (w237:bool)
    n138 = case shown="True" w237 {
      tunnel: w243 -> [_ w246]
      tunnel: w240 -> [_ w245]
      tunnel: w232 -> [_ w244]
      frame False {
      }
      frame True {
        n139 = call <vilib>:"Bind Controls to SmartDashboard.vi"("RPC ref"=w244, "Bound Control Refs"=w246, "Server IP Address"=w245) -> ()  [unwired: 9 in]
      }
    }
  }
  n140 = vi-ref "Playback Controls.vi"() -> (w64:refnum<vi>)
  n141 = property class="VI"() -> ("Panel"=w66:refnum<vi>)  [unwired: 2 in, 2 out]
  n142 = property class="Pnl"(reference=w66) -> ("Panes[]"=w67:refnum<vi>[])  [unwired: 1 in, 2 out]
  n143 = Index Array(array=w67) -> (element=w65:refnum<vi>)  [unwired: 1 in]
  n144 = control-ref of="Test Tree"() -> (w68:refnum<vi>)
  n145 = while {
    tunnel: [w256] -> _
    tunnel: w68 -> [w255]
    tunnel: w64 -> [w254]
    tunnel: w63 -> [w253]
    tunnel: w62 -> [_]
    tunnel: w58 -> [w252]
    tunnel: w25 -> [w251]
    tunnel: w23 -> [w250]
    shift-right: [w249] -> _
    shift-left: _ -> [w248]
    tunnel: w17 -> [w247]
    i -> [w256]
    stop <- FALSE stop-if-true
    n146 = event shown="[0] Timeout" {
      selector: w253 -> [_ _ _ _ _ _ _ _ _ _ _ _ _ _ _ _ _ _ _ _ _]
      dyn-events: [_ _ _ _ _ _ _ _ _ _ _ _ _ _ _ _ w516 _ _ _ _] -> _
      timeout: u32 60 ("milliseconds to wait") -> [_ _ _ _ _ _ _ _ _ _ _ _ _ _ _ _ _ _ _ _ _]
      tunnel: w255 -> [w268 _ _ _ _ _ _ _ _ _ _ _ _ _ _ _ _ _ _ _ _]
      tunnel: "Test Tree" -> [_ _ _ _ _ _ _ _ _ _ _ w483 w491 w493 w497 w505 _ _ _ _ _]
      tunnel: w254 -> [_ _ _ _ _ _ _ _ _ _ _ _ _ _ _ _ w518 _ w536 _ _]
      tunnel: w252 -> [_ _ _ _ _ _ _ _ _ _ _ _ _ _ _ _ w514 _ _ _ _]
      tunnel: w251 -> [_ _ _ _ _ _ _ _ _ _ _ _ _ _ _ _ w512 _ _ _ _]
      tunnel: w250 -> [w263 _ _ _ _ _ w434 _ _ _ _ _ _ _ _ _ _ _ _ _ _]
      tunnel: [w262 w311 w413 w418 w427 w431 w432 w441 w451 w458 w470 w482 w489 w492 w496 w504 w511 w531 w533 w537 w550] -> w249
      tunnel: w248 -> [w262 w311 w413 w418 w427 w431 w432 _ _ w458 w470 w482 w489 w492 w496 w504 w511 w531 w533 w537 w550]
      tunnel: w247 -> [w260 _ _ _ _ _ _ _ _ _ _ _ _ _ _ _ _ _ _ _ _]
      event Timeout {
        n147 = event-data() -> ()  [unwired: 1 in, 1 out]
        n148 = local read "Mode"() -> (w265:T4)
        n149 = case shown="\"Test\"" "Dashboard Tab" {
          tunnel: w268 -> [_ _ w284 _ _]
          tunnel: "TestMode/Automatic/" ("Name Pattern") -> [_ _ w283 _ _]
          tunnel: T22 [{"Operation"=enum."Clear", "Color Box"=14013909}, {"Operation"=enum."Clear", "Color Box"=14013909}, {"Operation"=enum."Clear", "Color Box"=14013909}, {"Operation"=enum."Clear", "Color Box"=14013909}, {"Operation"=enum."Update", "Color Box"=14013909}, {"Operation"=enum."Update", "Color Box"=16777215}, {"Operation"=enum."Clear", "Color Box"=14013909}, {"Operation"=enum."Clear", "Color Box"=14013909}, {"Operation"=enum."Clear", "Color Box"=14013909}] -> [_ _ w276 _ w304]
          tunnel: w265 -> [_ _ w275 _ w303]
          tunnel: u32[] [15790320, 15790320, 15790320, 15790320, 16777215, 16777215, 15790320, 15790320, 15790320] -> [_ _ _ _ w309]
          tunnel: w263 -> [_ _ _ _ w297]
          tunnel: w260 -> [_ w270 _ _ _]
          frame "Custom", Default {
          }
          frame "Basic" {
            n150 = call <vilib>:"WPI_DashboardUpdateNames.vi"("Controls on Tab"=w270) -> ()  [unwired: 11 in]
          }
          frame "Test" {
            w282 = -2 ("Active Item:Row Number")
            n151 = Index Array(array=w276, index=w275) -> (element=w277:T25)
            n152 = Unbundle(w277) -> ("Operation"=w278:enum16{"Update", "Clear"}, "Color Box"=w279:u32)
            n153 = call <vilib>:"NT Read String.vi"("Name"="TestMode/TestName") -> ("String"=w273:string)  [unwired: 9 in, 1 out]
            n154 = call <vilib>:"NT Read and Format Entries as Tree.vi"("Operation"=w278, "Name Pattern"=w283, "Tree Refnum"=w284) -> ()  [unwired: 7 in, 2 out]
            n155 = case shown="\"\"" w273 {
              tunnel: "TestMode/TestProgress" ("Name") -> [w286 _]
              tunnel: "TestMode/TestProgressText" ("Name") -> [w285 _]
              frame Default {
                n156 = call <vilib>:"NT Read Number.vi"("Name"=w286) -> ("Numeric"=w287:dbl)  [unwired: 9 in, 1 out]
                n157 = call <vilib>:"NT Read String.vi"("Name"=w285) -> ("String"=w288:string)  [unwired: 9 in, 1 out]
                n158 = Bundle("Numeric"=w287, "String"=w288) -> (→"Progress":cluster{"Numeric":dbl, "String":string})  [unwired: 1 in]
              }
              frame "" {
                n159 = property on="Progress" class="Clust (strict)"("Visible"=FALSE) -> ()  [unwired: 2 in, 2 out]
                n160 = local write "Test Name"(u16 0) -> ()
              }
            }
            n161 = property on="Test Tree" class="Tree (strict)"("Active Item Row Number"=w282, "ActiveColNum"=w282, "CellBG"=w279, "Active Item Row Number"=-1 ("Active Item:Row Number"), "CellBG"=u32 5789784 ("Color Box")) -> ()  [unwired: 2 in, 2 out]
          }
          frame "Variables" {
            w294 = string[] ["CameraPublisher", "Usage", "DB"]  # Items to initially close
            n162 = First Call?() -> (First Call?: T/F=w295:bool)
            n163 = control-ref of="Tree"() -> (w296:refnum<vi>)
            n164 = Select(t=w294, s=w295, f=string[] []) -> (s? t:f=w292:string[])
            n165 = call <vilib>:"NT Read and Format Entries as Tree.vi"("Tags to  Close"=w292, "Tree Refnum"=w296) -> ()  [unwired: 8 in, 2 out]
          }
          frame "Commands" {
            w305 = u32 5789784 ("Color Box")
            w306 = T26 {"Row"=-1, "Column"=-2} ("Active Cell:Active Cell")
            w308 = T26 {"Row"=-2, "Column"=-2} ("Active Cell:Active Cell")
            n166 = Index Array(array=w309, index=w303) -> (element=w307:u32)
            n167 = Index Array(array=w304, index=w303) -> (element=w302:T25)
            n168 = Unbundle(w302) -> ("Operation"=w301:enum16{"Update", "Clear"})  [unwired: 1 out]
            n169 = local read "Command Selection"() -> (w300:i32)
            n170 = property on="Command Selection" class="MCListbox (strict)"("ActiveCell"=w308, "CellBG"=w307, "ActiveCell"=w306, "CellBG"=w305) -> ()  [unwired: 2 in, 2 out]
            n171 = call <vilib>:"WPI_DashboardUpdate RPC Info.vi"("Operation"=w301) -> ("update"=w299:bool, "commands"=w298:string[][])  [unwired: 9 in]
            n172 = property on="Command Selection" class="MCListbox (strict)"("ItemNames"=w298) -> ()  [unwired: 2 in, 2 out]
            n173 = property on="Command Params" class="Tbl (strict)"("Active Cell"=w308, "Cell BG Color"=w307, "Active Cell"=w306, "Cell BG Color"=w305) -> ()  [unwired: 2 in, 2 out]
            n174 = call <vilib>:"WPI_DashboardUpdate Command Params.vi"("Update"=w299, "NewVal"=w300, "Commands"=w298, "Param Tbl"=w297) -> ()  [unwired: 7 in, 1 out]
          }
        }
        n175 = call <vilib>:"Connextion Info.vi"() -> ("Connected"=→"NT Connection":bool)  [unwired: 10 in, 1 out]
      }
      event "Test Tree": Value Change {
        # "Show appropriate\ncontrols"
        n176 = event-data() -> ("CtlRef"=w314:refnum<vi>, "NewVal"=w312:string)  [unwired: 1 in]
        n177 = call <vilib>:"WPI_UtilitiesGetTreeIOName.vi"("NewVal"=w312, "TreeControl in"=w314) -> ("I/O Name"=w315:string)  [unwired: 9 in]
        n178 = case shown="\"Camera\"" w315 {
          selector: w315 -> [_ w322 _ w344 w353 _]
          tunnel: w312 -> [_ _ w341 w343 _ w360]
          tunnel: cluster{string[]}[] [{["640x480", "320x240", "160x120"]}, {["Auto", "Fixed indoor", "Fixed outdoor 1", "Fixed outdoor 2", "Fixed fluorescent 1", "Fixed fluorescent 2", "Hold current"]}, {["Auto", "Flicker-free 50 Hz", "Flicker-free 60 Hz", "Hold current"]}, {["None", "Prioritize frame rate", "Prioritize image quality"]}, {["Monochrome", "Color"]}] -> [_ _ _ _ _ w359]
          frame Default {
            w317 = FALSE ("Visible")
            w316 = FALSE ("Visible")
            n179 = property on="Motor" class="Clust (strict)"("Visible"=w316) -> ()  [unwired: 2 in, 2 out]
            n180 = property on="Test Ring" class="Ring (strict)"("Visible"=w316) -> ()  [unwired: 2 in, 2 out]
            n181 = property on="Rev/Fwd" class="Clust (strict)"("Visible"=w317) -> ()  [unwired: 2 in, 2 out]
            n182 = property on="On/Off" class="Bool (strict)"("Visible"=w317) -> ()  [unwired: 2 in, 2 out]
            n183 = property on="Test Slider" class="Slide (strict)"("Visible"=w317) -> ()  [unwired: 2 in, 2 out]
          }
          frame "Analog Out", "Motor", "PWM" {
            w323 = FALSE ("Visible")
            n184 = case shown="\"Analog Out\"" w322 {
              tunnel: [1.0 ("Value") -1.0 ("Value") 0.0 ("Value")] -> w321
              tunnel: [255.0 ("Value") 1.0 ("Value") 5.0 ("Value")] -> w320
              tunnel: [128.0 ("Value") 0.0 ("Value") 0.0 ("Value")] -> w319
              tunnel: [64.0 ("Value") 0.5 ("Value") 1.0 ("Value")] -> w318
              frame "PWM" {
              }
              frame "Motor", Default {
              }
              frame "Analog Out" {
              }
            }
            n185 = property on="Motor" class="Clust (strict)"("Visible"=TRUE) -> ()  [unwired: 2 in, 2 out]
            n186 = property on="Value" class="Slide (strict)"("Value"=w319, "Scale.Minimum"=w321, "Scale.Maximum"=w320, "Scale.Increment"=w318) -> ()  [unwired: 2 in, 2 out]
            n187 = property on="On/Off" class="Bool (strict)"("Visible"=w323) -> ()  [unwired: 2 in, 2 out]
            n188 = property on="Test Slider" class="Slide (strict)"("Visible"=w323) -> ()  [unwired: 2 in, 2 out]
            n189 = property on="Test Ring" class="Ring (strict)"("Visible"=w323) -> ()  [unwired: 2 in, 2 out]
            n190 = property on="Rev/Fwd" class="Clust (strict)"("Visible"=w323) -> ()  [unwired: 2 in, 2 out]
          }
          frame "Servo" {
            w339 = FALSE ("Visible")
            n191 = call <vilib>:"NT Read Number.vi"("Name"=w341) -> ("Numeric"=w340:dbl)  [unwired: 9 in, 1 out]
            n192 = property on="Test Slider" class="Slide (strict)"("Visible"=TRUE, "Scale.Maximum"=170.0 ("Scale.Range:Maximum")) -> ()  [unwired: 2 in, 2 out]
            n193 = local write "Test Slider"(w340) -> ()
            n194 = property on="Motor" class="Clust (strict)"("Visible"=w339) -> ()  [unwired: 2 in, 2 out]
            n195 = property on="Rev/Fwd" class="Clust (strict)"("Visible"=w339) -> ()  [unwired: 2 in, 2 out]
            n196 = property on="On/Off" class="Bool (strict)"("Visible"=w339) -> ()  [unwired: 2 in, 2 out]
            n197 = property on="Test Ring" class="Ring (strict)"("Visible"=w339) -> ()  [unwired: 2 in, 2 out]
          }
          frame "Relay", "Solenoid" {
            w342 = FALSE ("Visible")
            n198 = property on="Motor" class="Clust (strict)"("Visible"=w342) -> ()  [unwired: 2 in, 2 out]
            n199 = property on="Test Slider" class="Slide (strict)"("Visible"=w342) -> ()  [unwired: 2 in, 2 out]
            n200 = Search and Replace String(input string=w343, search string="/Value  **", replace string="/Direction") -> (result string=w349:string)  [unwired: 5 in, 3 out]
            n201 = property on="Test Ring" class="Ring (strict)"("Visible"=w342) -> ()  [unwired: 2 in, 2 out]
            n202 = call <vilib>:"NT Read String.vi"("Name"=w349) -> ("String"=w347:string)  [unwired: 9 in, 1 out]
            n203 = Equal?(x="Both directions", y=w347) -> (x = y?=w345:bool)
            n204 = Not(x=w345) -> (.not. x?=w346:bool)
            n205 = property on="Rev/Fwd" class="Clust (strict)"("Visible"=w345) -> ()  [unwired: 2 in, 2 out]
            n206 = property on="On/Off" class="Bool (strict)"("Visible"=w346, "Caption.Text"=w344) -> ()  [unwired: 2 in, 2 out]
          }
          frame "Compressor", "Digital Out" {
            w352 = FALSE ("Visible")
            # "Get direction and finish"
            n207 = property on="Motor" class="Clust (strict)"("Visible"=w352) -> ()  [unwired: 2 in, 2 out]
            n208 = property on="Test Slider" class="Slide (strict)"("Visible"=w352) -> ()  [unwired: 2 in, 2 out]
            n209 = property on="Test Ring" class="Ring (strict)"("Visible"=w352) -> ()  [unwired: 2 in, 2 out]
            n210 = property on="On/Off" class="Bool (strict)"("Visible"=TRUE, "Caption.Text"=w353) -> ()  [unwired: 2 in, 2 out]
            n211 = property on="Rev/Fwd" class="Clust (strict)"("Visible"=FALSE) -> ()  [unwired: 2 in, 2 out]
          }
          frame "Camera" {
            n212 = call <vilib>:"Get Last Path Segment.vi"("String in"=w360) -> ("String out"=w361:string)  [unwired: 10 in]
            n213 = property on="On/Off" class="Bool (strict)"("Visible"=FALSE) -> ()  [unwired: 2 in, 2 out]
            n214 = property on="Motor" class="Clust (strict)"("Visible"=FALSE) -> ()  [unwired: 2 in, 2 out]
            n215 = property on="Rev/Fwd" class="Clust (strict)"("Visible"=FALSE) -> ()  [unwired: 2 in, 2 out]
            n216 = case shown="\"White Balance  **\"" w361 {
              tunnel: w360 -> [w367 w376 w385 w394 w403 _ w409]
              tunnel: w359 -> [w365 w373 w382 w391 w400 _ _]
              frame "Size  **" {
                n217 = Index Array(array=w365) -> (element=w364:cluster{string[]})  [unwired: 1 in]
                n218 = call <vilib>:"NT Read String.vi"("Name"=w367) -> ("String"=w366:string)  [unwired: 9 in, 1 out]
                n219 = Unbundle(w364) -> (w362:string[])
                n220 = Match First String(2:w362, 3:w366) -> (0:w363:i32)  [unwired: 1 out]
                n221 = property on="Test Ring" class="Ring (strict)"("Value"=w363, "Strings []"=w362) -> ()  [unwired: 2 in, 2 out]
                n222 = property on="Test Ring" class="Ring (strict)"("Visible"=TRUE) -> ()  [unwired: 2 in, 2 out]
                n223 = property on="Test Slider" class="Slide (strict)"("Visible"=FALSE) -> ()  [unwired: 2 in, 2 out]
              }
              frame "White Balance  **" {
                n224 = Index Array(array=w373, index=1) -> (element=w374:cluster{string[]})
                n225 = call <vilib>:"NT Read String.vi"("Name"=w376) -> ("String"=w375:string)  [unwired: 9 in, 1 out]
                n226 = Unbundle(w374) -> (w371:string[])
                n227 = Match First String(2:w371, 3:w375) -> (0:w370:i32)  [unwired: 1 out]
                n228 = property on="Test Ring" class="Ring (strict)"("Value"=w370, "Strings []"=w371) -> ()  [unwired: 2 in, 2 out]
                n229 = property on="Test Ring" class="Ring (strict)"("Visible"=TRUE) -> ()  [unwired: 2 in, 2 out]
                n230 = property on="Test Slider" class="Slide (strict)"("Visible"=FALSE) -> ()  [unwired: 2 in, 2 out]
              }
              frame "Exposure  **" {
                n231 = Index Array(array=w382, index=2) -> (element=w383:cluster{string[]})
                n232 = call <vilib>:"NT Read String.vi"("Name"=w385) -> ("String"=w384:string)  [unwired: 9 in, 1 out]
                n233 = Unbundle(w383) -> (w379:string[])
                n234 = Match First String(2:w379, 3:w384) -> (0:w380:i32)  [unwired: 1 out]
                n235 = property on="Test Ring" class="Ring (strict)"("Value"=w380, "Strings []"=w379) -> ()  [unwired: 2 in, 2 out]
                n236 = property on="Test Ring" class="Ring (strict)"("Visible"=TRUE) -> ()  [unwired: 2 in, 2 out]
                n237 = property on="Test Slider" class="Slide (strict)"("Visible"=FALSE) -> ()  [unwired: 2 in, 2 out]
              }
              frame "Exposure Priority  **" {
                n238 = Index Array(array=w391, index=3) -> (element=w392:cluster{string[]})
                n239 = call <vilib>:"NT Read String.vi"("Name"=w394) -> ("String"=w393:string)  [unwired: 9 in, 1 out]
                n240 = Unbundle(w392) -> (w388:string[])
                n241 = Match First String(2:w388, 3:w393) -> (0:w389:i32)  [unwired: 1 out]
                n242 = property on="Test Ring" class="Ring (strict)"("Value"=w389, "Strings []"=w388) -> ()  [unwired: 2 in, 2 out]
                n243 = property on="Test Ring" class="Ring (strict)"("Visible"=TRUE) -> ()  [unwired: 2 in, 2 out]
                n244 = property on="Test Slider" class="Slide (strict)"("Visible"=FALSE) -> ()  [unwired: 2 in, 2 out]
              }
              frame "Color Enable  **" {
                n245 = Index Array(array=w400, index=4) -> (element=w401:cluster{string[]})
                n246 = call <vilib>:"NT Read String.vi"("Name"=w403) -> ("String"=w402:string)  [unwired: 9 in, 1 out]
                n247 = Unbundle(w401) -> (w397:string[])
                n248 = Match First String(2:w397, 3:w402) -> (0:w398:i32)  [unwired: 1 out]
                n249 = property on="Test Ring" class="Ring (strict)"("Value"=w398, "Strings []"=w397) -> ()  [unwired: 2 in, 2 out]
                n250 = property on="Test Ring" class="Ring (strict)"("Visible"=TRUE) -> ()  [unwired: 2 in, 2 out]
                n251 = property on="Test Slider" class="Slide (strict)"("Visible"=FALSE) -> ()  [unwired: 2 in, 2 out]
              }
              frame Default {
                n252 = property on="Test Ring" class="Ring (strict)"("Visible"=FALSE) -> ()  [unwired: 2 in, 2 out]
                n253 = property on="Test Slider" class="Slide (strict)"("Visible"=FALSE) -> ()  [unwired: 2 in, 2 out]
              }
              frame "Brightness  **", "Color Level  **", "Compression  **", "FPS  **", "Sharpness  **" {
                n254 = call <vilib>:"NT Read Number.vi"("Name"=w409) -> ("Numeric"=w408:dbl)  [unwired: 9 in, 1 out]
                n255 = local write "Test Slider"(w408) -> ()
                n256 = property on="Test Slider" class="Slide (strict)"("Visible"=TRUE, "Scale.Maximum"=100.0 ("Scale.Range:Maximum")) -> ()  [unwired: 2 in, 2 out]
                n257 = property on="Test Ring" class="Ring (strict)"("Visible"=FALSE) -> ()  [unwired: 2 in, 2 out]
              }
            }
          }
        }
        n258 = property on="Progress" class="Clust (strict)"("Visible"=FALSE) -> ()  [unwired: 2 in, 2 out]
      }
      event "Test Name": Mouse Enter {
        # "Populate the ring with the list of tests"
        n259 = event-data() -> ()  [unwired: 1 in, 1 out]
        n260 = call <vilib>:"NT Read String Array.vi"("Name"="TestMode/TestList") -> ("String Array"=w417:string[])  [unwired: 9 in, 1 out]
        n261 = Build Array (concatenate)("Select the test to run...", w417) -> (w416:string[])
        n262 = property on="Test Name" class="Ring (strict)"("Strings []"=w416) -> ()  [unwired: 2 in, 2 out]
      }
      event "Test Name": Value Change {
        w419 = FALSE ("Visible")
        # "Tell the robot the test name to run"
        n263 = event-data() -> ("NewVal"=w423:u16)  [unwired: 1 in]
        n264 = property on="Test Name" class="Ring (strict)"() -> ("Strings []"=w424:string[])  [unwired: 2 in, 2 out]
        n265 = local write "Progress"(T6 {"Test Progress"=0, "Test Progress Text"=""} ("Progress")) -> ()
        n266 = Index Array(array=w424, index=w423) -> (element=w422:string)
        n267 = call <vilib>:"NT Write String.vi"("String"=w422, "Name"="TestMode/TestName") -> ()  [unwired: 9 in, 1 out]
        n268 = property on="Progress" class="Clust (strict)"("Visible"=TRUE) -> ()  [unwired: 2 in, 2 out]
        n269 = property on="Motor" class="Clust (strict)"("Visible"=w419) -> ()  [unwired: 2 in, 2 out]
        n270 = property on="Test Slider" class="Slide (strict)"("Visible"=w419) -> ()  [unwired: 2 in, 2 out]
        n271 = property on="On/Off" class="Bool (strict)"("Visible"=w419) -> ()  [unwired: 2 in, 2 out]
        n272 = property on="Rev/Fwd" class="Clust (strict)"("Visible"=w419) -> ()  [unwired: 2 in, 2 out]
        n273 = property on="Test Ring" class="Ring (strict)"("Visible"=w419) -> ()  [unwired: 2 in, 2 out]
      }
      event "Select Auto": Mouse Enter {
        # "Populate the combo box with the list of autonomous options"
        n274 = event-data() -> ()  [unwired: 1 in, 1 out]
        n275 = call <vilib>:"NT Read String Array.vi"("Name"="Auto List") -> ("String Array"=w426:string[])  [unwired: 9 in, 1 out]
        n276 = property on="Select Auto" class="CmbBox"("Strings[]"=w426) -> ()  [unwired: 2 in, 2 out]
      }
      event "Select Auto": Value Change {
        # "User modified the Auto Selection. Write to NT variable so robot knows."
        n277 = event-data() -> ("NewVal"=w429:string)  [unwired: 1 in]
        n278 = call <vilib>:"NT Write String.vi"("String"=w429, "Name"="Auto Selector") -> ()  [unwired: 9 in, 1 out]
      }
      event "Command Selection": Value Change {
        # "Get the params and show in table"
        n279 = event-data() -> ("NewVal"=w435:i32)  [unwired: 1 in]
        n280 = property on="Command Selection" class="MCListbox (strict)"() -> ("ItemNames"=w433:string[][])  [unwired: 2 in, 2 out]
        n281 = call <vilib>:"WPI_DashboardUpdate Command Params.vi"("NewVal"=w435, "Commands"=w433, "Param Tbl"=w434) -> ()  [unwired: 8 in, 1 out]
      }
      event "Execute Command": Value Change {
        # "Started one, Unique ID holds\nresponse"
        n282 = event-data() -> ()  [unwired: 1 in, 1 out]
        n283 = property on="Command Selection" class="MCListbox (strict)"() -> ("ItemNames"=w446:string[][])  [unwired: 2 in, 2 out]
        n284 = Index Array(array=w446, index (row)="Command Selection", index (col)=0) -> (element=w444:string)
        n285 = call <vilib>:"Invoke Commands.vi"("Command Params"="Command Params", "Function Name"=w444) -> ("Params"=w440:u8, "Started"=w439:bool)  [unwired: 7 in, 1 out]
        n286 = Array Subset(array="Command Params", length (row)=w440) -> (w441:string[][])  [unwired: 3 in]
        n287 = Select(t="Executing" ("Cmd Status"), s=w439, f="" ("Cmd Status")) -> (s? t:f=→"Cmd Status":string)
      }
      event "Command Selection": Double Click {
        n288 = event-data() -> ("Row"=w454:i32)  [unwired: 1 in]
        n289 = property on="Command Selection" class="MCListbox (strict)"() -> ("ItemNames"=w457:string[][])  [unwired: 2 in, 2 out]
        n290 = local read "Command Params"() -> (w453:string[][])
        n291 = Index Array(array=w457, index (row)=w454, index (col)=0) -> (element=w455:string)
        n292 = call <vilib>:"Invoke Commands.vi"("Command Params"=w453, "Function Name"=w455) -> ("Params"=w452:u8, "Started"=w447:bool)  [unwired: 7 in, 1 out]
        n293 = Array Subset(array=w453, length (row)=w452) -> (w451:string[][])  [unwired: 3 in]
        n294 = Select(t="Executing" ("Cmd Status"), s=w447, f="" ("Cmd Status")) -> (s? t:f=w448:string)
        n295 = local write "Cmd Status"(w448) -> ()
      }
      event "CheckList": Double Click {
        # "Shift clears all"
        # "Update symbols on the listbox"
        n296 = event-data() -> ("PlatMods.Shift"=w459:bool, "Row"=w461:i32)  [unwired: 1 in]
        n297 = case shown="True" w459 {
          tunnel: w461 -> [w465 _]
          tunnel: 1 -> [w464 _]
          frame False {
            n298 = property on="CheckList" class="LstBox (strict)"() -> ("Item Symbols"=w463:i32[])  [unwired: 2 in, 2 out]
            n299 = Replace Array Subset(array=w463, new element=w464, index=w465) -> (w462:i32[])
            n300 = property on="CheckList" class="LstBox (strict)"("Item Symbols"=w462) -> ()  [unwired: 2 in, 2 out]
          }
          frame True {
            w466 = 0 ("Top Row")
            n301 = property on="CheckList" class="LstBox (strict)"() -> ("Number of Rows"=w468:u32)  [unwired: 2 in, 2 out]
            n302 = Initialize Array(0, w468) -> (w467:i32[])
            n303 = property on="CheckList" class="LstBox (strict)"("Top Row"=w466, "Value"=w466, "Item Symbols"=w467) -> ()  [unwired: 2 in, 2 out]
          }
        }
      }
      event "CheckList": Key Down {
        # "Update symbols on the listbox\nLeft and right keys check and uncheck"
        n304 = event-data() -> ("VKey"=w472:T23)  [unwired: 1 in]
        n305 = case shown="\"Left\", \"Right\"" w472 {
          selector: w472 -> [w477 _]
          tunnel: eventvkey."Left" ("VKey") -> [w475 _]
          frame "Left", "Right" {
            n306 = Equal?(x=w475, y=w477) -> (x = y?=w476:bool)
            n307 = Select(t=0, s=w476, f=1) -> (s? t:f=w478:i32)
            n308 = property on="CheckList" class="LstBox (strict)"() -> ("Item Symbols"=w481:i32[])  [unwired: 2 in, 2 out]
            n309 = Replace Array Subset(array=w481, new element=w478, index="CheckList") -> (w480:i32[])
            n310 = property on="CheckList" class="LstBox (strict)"("Item Symbols"=w480) -> ()  [unwired: 2 in, 2 out]
          }
          frame Default {
          }
        }
      }
      event "Motor.Enable": Value Change {
        # "When the test mode otor enable helper is set, update that\ntree row item's value"
        n311 = event-data() -> ("NewVal"=w487:bool)  [unwired: 1 in]
        n312 = Unbundle("Motor") -> ("Value"=w486:dbl)  [unwired: 1 out]
        n313 = Select(t=w486, s=w487, f=0.0) -> (s? t:f=w484:dbl)
        n314 = call <vilib>:"NT Write Number.vi"("Numeric"=w484, "Name"=w483) -> ()  [unwired: 9 in, 1 out]
      }
      event "Test Slider": Value Change {
        # "When the test mode slider helper is set, update that\ntree row item's value"
        n315 = event-data() -> ("NewVal"=w490:dbl)  [unwired: 1 in]
        n316 = call <vilib>:"NT Write Number.vi"("Numeric"=w490, "Name"=w491) -> ()  [unwired: 9 in, 1 out]
      }
      event "On/Off": Value Change {
        # "When the test mode on/off helper value is set, update that\ntree row item's value"
        n317 = event-data() -> ("NewVal"=w495:bool)  [unwired: 1 in]
        n318 = Boolean To (0,1)(Boolean=w495) -> (0, 1=w494:i16)
        n319 = call <vilib>:"NT Write Number.vi"("Numeric"=w494, "Name"=w493) -> ()  [unwired: 9 in, 1 out]
      }
      event "Rev/Fwd": Value Change {
        # "When the test mode helper value for relays is set, update that\ntree row item's value"
        n320 = event-data() -> ("NewVal.Forward"=w503:bool, "NewVal.Reverse"=w502:bool)  [unwired: 1 in]
        n321 = Boolean To (0,1)(Boolean=w503) -> (0, 1=w499:i16)
        n322 = Boolean To (0,1)(Boolean=w502) -> (0, 1=w501:i16)
        n323 = Negate(x=w501) -> (-x=w500:i16)
        n324 = Add(x=w499, y=w500) -> (x+y=w498:i16)
        n325 = call <vilib>:"NT Write Number.vi"("Numeric"=w498, "Name"=w497) -> ()  [unwired: 9 in, 1 out]
      }
      event "Test Ring": Value Change {
        # "When a test mode helper value is selected from the ring,\nset the tree item's variable to the string value"
        n326 = event-data() -> ("NewVal"=w507:u16)  [unwired: 1 in]
        n327 = property on="Test Ring" class="Ring (strict)"() -> ("Strings []"=w508:string[])  [unwired: 2 in, 2 out]
        n328 = Index Array(array=w508, index=w507) -> (element=w506:string)
        n329 = call <vilib>:"NT Write String.vi"("String"=w506, "Name"=w505) -> ()  [unwired: 9 in, 1 out]
      }
      event "Rec Mode": Value Change {
        # "Update globals for recording mode and path to read log from.\nClear when logging and let NetworkTables set path for vision to\nuse."
        n330 = event-data() -> ("NewVal"=w519:enum32{"Stop", "Record", "Playback"})  [unwired: 1 in]
        n331 = global write "WPI_DashboardLogging Global.vi" "Logging Filename"(path "") -> ()
        n332 = global write "WPI_DashboardLogging Global.vi" "Recording"(w519) -> ()
        n333 = case shown="\"Playback\"" w519 {
          tunnel: w518 -> [_ w521 w530]
          tunnel: [_ _ w529] -> w516
          tunnel: [_ _ w528] -> _
          tunnel: w514 -> [_ _ w526]
          tunnel: cluster{i32, i32} {-250, 170} -> [_ _ w525]
          tunnel: [_ _ T24 {"Image Size"=TRUE, "Image Type"=TRUE, "Pixel Value"=TRUE, "ROI Information"=TRUE, "Zoom Factor"=FALSE} ("Image Information Shown:All Elements")] -> w509
          tunnel: [_ _ TRUE ("Zoom Factor")] -> w510
          tunnel: w512 -> [_ _ w522]
          frame Default {
          }
          frame "Stop", "Record" {
            # "Place Window too"
            n334 = invoke class="VI" method="FP.Close"(reference=w521) -> (reference out=w520:refnum<vi>)  [unwired: 2 in, 2 out]
            n335 = invoke class="VI" method="Abort VI"(reference=w520) -> ()  [unwired: 2 in, 3 out]
          }
          frame "Playback" {
            n336 = call "Open Playback Panel.vi"("Offset"=w525, "DB VI Ref"=w526, "Playback in"=w530) -> ("Playback out"=w527:refnum<vi>)  [unwired: 8 in]
            n337 = register-events(w527, w522) -> (reference out=w529:refnum<event-registration>, error out=w528:errorcluster)  [unwired: 2 in]
          }
        }
        n338 = property on="Camera Image Right" class="ImageControl"("Image Information Shown"=w509, "Image Information Visible"=w510) -> ()  [unwired: 2 in, 2 out]
        n339 = property on="Camera Image" class="ImageControl"("Image Information Shown"=w509, "Image Information Visible"=w510) -> ()  [unwired: 2 in, 2 out]
        n340 = call <vilib>:"WPI_DashboardNT Log FieldName Cache.vi"("Operation"=enum16{"Lookup/Add", "Index", "Clear"}."Clear") -> ()  [unwired: 8 in, 3 out]
      }
      event Panel Close {
        w532 = enum32{"Stop", "Record", "Playback"}."Stop" ("Rec Mode")
        # "Playback window has been closed, abort"
        n341 = event-data() -> ()  [unwired: 1 in, 4 out]
        n342 = local write "Rec Mode"(w532) -> ()
        n343 = global write "WPI_DashboardLogging Global.vi" "Recording"(w532) -> ()
      }
      event Panel Close {
        # "Abort playback window and ourself"
        n344 = event-data() -> ()  [unwired: 1 in, 4 out]
        n345 = invoke class="VI" method="FP.Close"(reference=w536) -> (reference out=w535:refnum<vi>)  [unwired: 2 in, 2 out]
        n346 = invoke class="VI" method="Abort VI"(reference=w535) -> (error out=w534:errorcluster)  [unwired: 2 in, 2 out]
        n347 = invoke class="VI" method="Abort VI"(error in=w534) -> ()  [unwired: 2 in, 3 out]
      }
      event User Event {
        n348 = event-data() -> ("IDs"=w543:cluster{"RPC field ID":u16, "Unique ID":u16}, "String"=w542:string)  [unwired: 1 in]
        n349 = Bundle("IDs"=w543, "String"=w542) -> (w541:T9)  [unwired: 1 in]
        n350 = call <vilib>:"Retrieve RPC Response.vi"("RPC Response"=w541) -> ("Output"=w539:string[][])  [unwired: 10 in]
        n351 = Build Array (concatenate)(w537, w539) -> (w538:string[][])
        n352 = local write "Command Params"(w538) -> ()
        n353 = local write "Cmd Status"("" ("Cmd Status")) -> ()
      }
      event "Tree": Double Click {
        n354 = event-data() -> ("PlatMods"=w549:T27, "Tag"=w546:string)  [unwired: 1 in]
        n355 = Unbundle(w549) -> ("Shift"=w548:bool)  [unwired: 4 out]
        n356 = String Subset(string=w546, length (rest)=1 ("length (rest)")) -> (substring=w545:string)  [unwired: 1 in]
        n357 = Not(x=w548) -> (.not. x?=w547:bool)
        n358 = case shown="\"/\"" w545 {
          tunnel: w546 -> [_ w552]
          tunnel: w547 -> [_ w551]
          frame Default {
          }
          frame "/" {
            n359 = call <vilib>:"NT Update Persistence.vi"("Persistence"=w551, "Name"=w552) -> ()  [unwired: 9 in, 1 out]
          }
        }
      }
    }
  }
  n360 = while {
    tunnel: w65 -> [w554]
    i -> [w557]
    stop <- FALSE stop-if-true
    n361 = Wait (ms)(milliseconds to wait=u32 100) -> ()  [unwired: 1 out]
    n362 = case shown="\"Playback\"" "Rec Mode" {
      tunnel: w557 -> [_ _ w572]
      tunnel: [u32 2829099 ("Base Color") u32 11141120 ("Target Color") w561] -> w553
      frame "Stop", Default {
        # "Reset the color, extra updates don't cost much"
      }
      frame "Record" {
      }
      frame "Playback" {
        # "Playback"
        n363 = Quotient & Remainder(x=w572, y=u32 50 ("milliseconds to wait")) -> (x-y*floor(x/y)=w568:u32)  [unwired: 1 out]
        n364 = Divide(x=w568, y=u32 50 ("milliseconds to wait")) -> (x/y=w565:dbl)
        n365 = Multiply(x=6.283185307179586, y=w565) -> (x*y=w570:dbl)
        n366 = Sine(x=w570) -> (sin(x)=w569:dbl)
        n367 = Absolute Value(x=w569) -> (abs(x)=w562:dbl)
        n368 = call "Interpolate RGB Color.vi"("Proportion"=w562, "Target Color"=u32 30976, "Base Color"=u32 2829099) -> ("Result Color"=w561:u32)  [unwired: 8 in]
      }
    }
    n369 = property class="Pane"(reference=w554, "PaneColor"=w553) -> ()  [unwired: 1 in, 2 out]
  }
  n370 = local write "Dashboard Tab"(T2."Drive" ("Dashboard Tab")) -> ()
  n371 = property on="On/Off" class="Bool (strict)"("Visible"=w36) -> ()  [unwired: 2 in, 2 out]
  n372 = property on="Motor" class="Clust (strict)"("Visible"=w36) -> ()  [unwired: 2 in, 2 out]
  n373 = property on="Progress" class="Clust (strict)"("Visible"=w36) -> ()  [unwired: 2 in, 2 out]
  n374 = property on="Test Ring" class="Ring (strict)"("Visible"=w36) -> ()  [unwired: 2 in, 2 out]
  n375 = property on="Rev/Fwd" class="Clust (strict)"("Visible"=w36) -> ()  [unwired: 2 in, 2 out]
  n376 = while {
    tunnel: u16 1741 ("timeout ms (25000)") -> [w574]
    stop <- FALSE stop-if-true
    n377 = TCP Create Listener(10:w574) -> (0:w573:errorcluster, 3:w575:refnum<k5>)  [unwired: 4 in, 1 out]
    n378 = case shown="No Error" w573 {
      selector: w573 -> [w577 _]
      tunnel: w575 -> [w578 _]
      frame No Error {
        n379 = while {
          tunnel: w578 -> [w581]
          tunnel: w577 -> [w580]
          stop <- FALSE stop-if-true
          n380 = TCP Wait On Listener(8:w580, 11:w581) -> (0:w582:errorcluster, 4:w583:refnum<k5>)  [unwired: 2 in, 3 out]
          n381 = local write "TCP"(w583) -> ()
          n382 = case shown="No Error" w582 {
            frame No Error {
            }
            frame Error {
              n383 = Wait (ms)(milliseconds to wait=u32 1000) -> ()  [unwired: 1 out]
            }
          }
        }
      }
      frame Error {
        n384 = Wait (ms)(milliseconds to wait=u32 1000) -> ()  [unwired: 1 out]
      }
    }
  }
  n385 = local write "Command Selection"(u16 0 ("milliseconds to wait")) -> ()
  n386 = local write "Command Params"(string[][] [] ("Command Params")) -> ()
  n387 = global write "WPI_DashboardLogging Global.vi" "Recording"(w59) -> ()
  n388 = local write "Rec Mode"(w59) -> ()
  n389 = call <vilib>:"NT Write String.vi"("String"="Select Auto", "Name"="Auto Selector") -> ()  [unwired: 9 in, 1 out]
